vi "prompt_with_timeout_launcher_v2.0.vi"(8 "error in (no error)":errorcluster, 9 "blink_timer(sec)":dbl=0.5, 10 "timer(sec)":dbl=3.0, 11 "message in":string="Not valid to run the test..") -> (0 "error out":errorcluster)   [LabVIEW 2025]
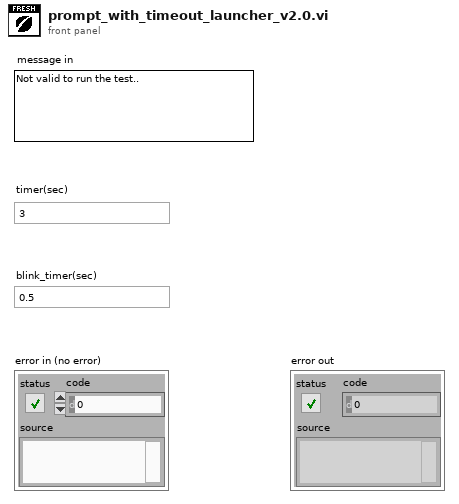
[diagram p1: front panel]
types:
  T1 = enum32{"Bad", "Idle", "Run top level", "Running"}
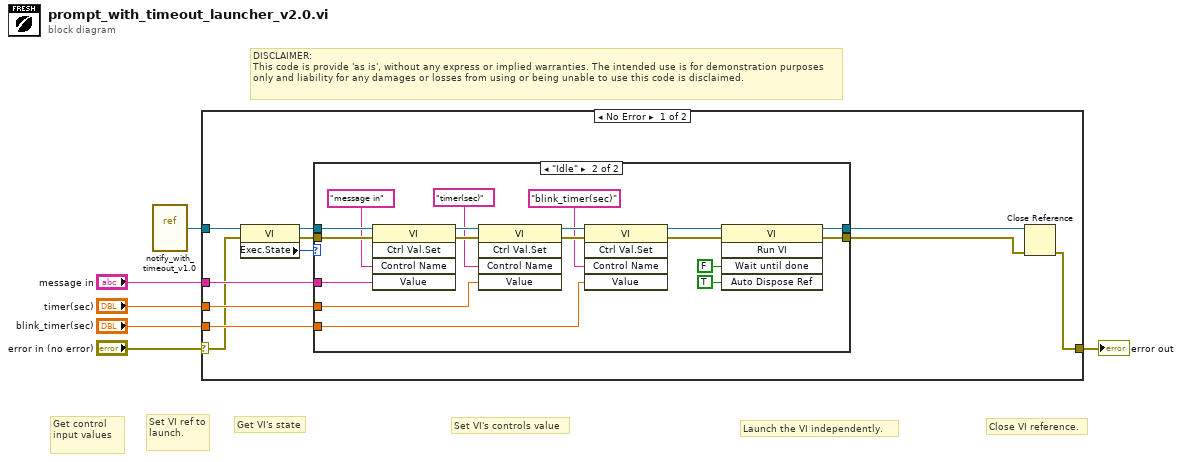
[diagram p0: block diagram]
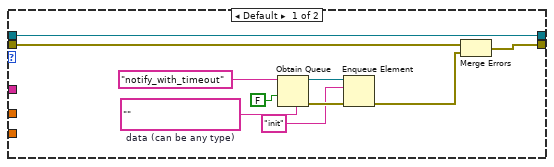
[diagram p2: hidden frame]
diagram:
  # "Close VI reference."
  # "Launch the VI independently."
  # "Set VI's controls value"
  # "Get VI's state"
  # "Set VI ref to launch."
  # "Get control input values"
  # "DISCLAIMER:\nThis code is provide 'as is', without any express or implied warranties. The intended use is for demonstration purposes only and liability for any damages or losses from using or being unable to use this code is disclaimed."
  n1 = vi-ref "notify_with_timeout_v1.0.vi"() -> (w6:refnum<vi>)
  n2 = case shown="No Error" "error in (no error)" {
    selector: "error in (no error)" -> [w10 w46]
    tunnel: w6 -> [w9 _]
    tunnel: [w14 w46] -> w4
    tunnel: "message in" -> [w13 _]
    tunnel: "timer(sec)" -> [w12 _]
    tunnel: "blink_timer(sec)" -> [w11 _]
    frame No Error {
      n3 = property class="VI"(reference=w9, error in=w10) -> (reference out=w16:refnum<vi>, error out=w15:errorcluster, "Exec.State"=w17:T1)
      n4 = case shown="\"Idle\"" w17 {
        tunnel: w16 -> [w26 w39]
        tunnel: w15 -> [w27 w43]
        tunnel: [w26 w29] -> w7
        tunnel: [w19 w28] -> w8
        tunnel: w13 -> [_ w32]
        tunnel: w12 -> [_ w31]
        tunnel: w11 -> [_ w30]
        frame Default {
          w25 = ""  # data (can be any type)
          n5 = Obtain Queue(name (unnamed)="notify_with_timeout", element data type=w25, create if not found? (T)=FALSE) -> (queue out=w22:refnum<queue>, error out=w23:errorcluster)  [unwired: 2 in, 1 out]
          n6 = Enqueue Element(queue=w22, element="init", error in (no error)=w23) -> (error out=w18:errorcluster)  [unwired: 1 in, 2 out]
          n7 = Merge Errors(w27, w18) -> (w19:errorcluster)
        }
        frame "Idle" {
          n8 = invoke class="VI" method="Ctrl Val.Set"(reference=w39, error in=w43, "Control Name"="message in", "Value"=w32) -> (reference out=w38:refnum<vi>, error out=w42:errorcluster)  [unwired: 1 in, 3 out]
          n9 = invoke class="VI" method="Ctrl Val.Set"(reference=w38, error in=w42, "Control Name"="timer(sec)", "Value"=w31) -> (reference out=w37:refnum<vi>, error out=w41:errorcluster)  [unwired: 1 in, 3 out]
          n10 = invoke class="VI" method="Ctrl Val.Set"(reference=w37, error in=w41, "Control Name"="blink_timer(sec)", "Value"=w30) -> (reference out=w36:refnum<vi>, error out=w40:errorcluster)  [unwired: 1 in, 3 out]
          n11 = invoke class="VI" method="Run VI"(reference=w36, error in=w40, "Wait until done"=FALSE ("Wait Until Done"), "Auto Dispose Ref"=TRUE ("Auto Dispose Reference")) -> (reference out=w29:refnum<vi>, error out=w28:errorcluster)  [unwired: 1 in, 3 out]
        }
      }
      n12 = Close Reference(reference=w7, error in (no error)=w8) -> (error out=w14:errorcluster)
    }
    frame Error {
    }
  }
  "error out" <- w4
